vi "VI Copier.vi"(8 "error in":errorcluster, 11 "Source Path":path) -> (0 "error out":errorcluster, 3 "Copy Path":path)   [LabVIEW 2011]
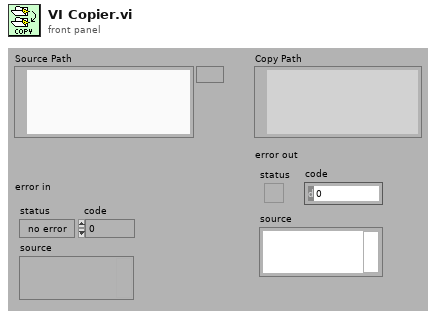
[diagram p1: front panel]
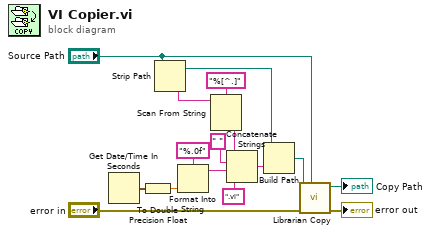
[diagram p0: block diagram]
diagram:
  n1 = Get Date/Time In Seconds() -> (seconds since 1Jan1904=w4:timestamp)
  n2 = To Double Precision Float(number=w4) -> (double precision float=w3:dbl)
  n3 = Strip Path(path="Source Path") -> (stripped path=w8:path, name=w6:string)
  n4 = Format Into String(format string="%.0f", w3) -> (resulting string=w1:string)  [unwired: 2 in, 1 out]
  n5 = Scan From String(format string="%[^.]", input string=w6) -> (output 1=w5:string)  [unwired: 2 in, 4 out]
  n6 = Concatenate Strings(w5, " " ("string"), w1, ".vi" ("string")) -> (w11:string)
  n7 = Build Path(base path=w8, name or relative path=w11) -> (appended path=w10:path)
  n8 = call <vilib>:"Librarian Copy.vi"("source"="Source Path", "error in (no error)"="error in", "destination"=w10) -> ("error out"=→"error out":errorcluster, "dup destination"=→"Copy Path":path)  [unwired: 2 in, 5 out]
